vi "Init.vi"(8 "error in (no error)":errorcluster, 11 "Process In":refnum<class "Process.lvclass">) -> (0 "error out":errorcluster, 3 "Process Out":refnum<class "Process.lvclass">)   [LabVIEW 2020, in "Process.lvclass"]
doc: "Initializes the process and creates necessary references. Anything initialized here is released in the Clear.vi method."
uses:
  Process.lvclass
  Protected/Message Cluster.ctl
  Process.lvclass/Process.ctl
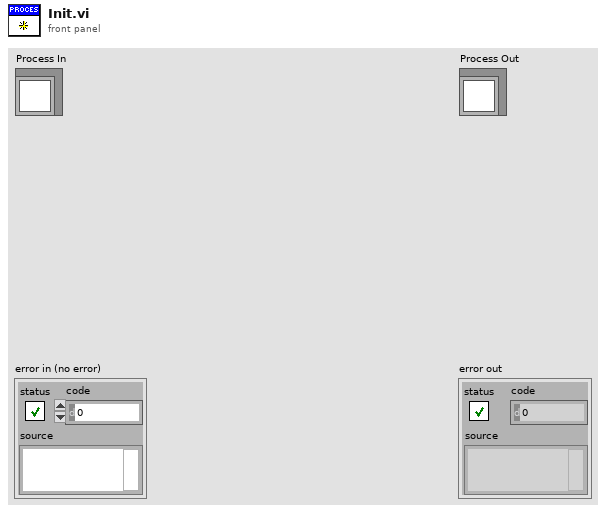
[diagram p1: front panel]
types:
  T1 = typedef "Process.lvclass/Message Cluster.ctl" = cluster{"Message":string, "Message Data":variant}
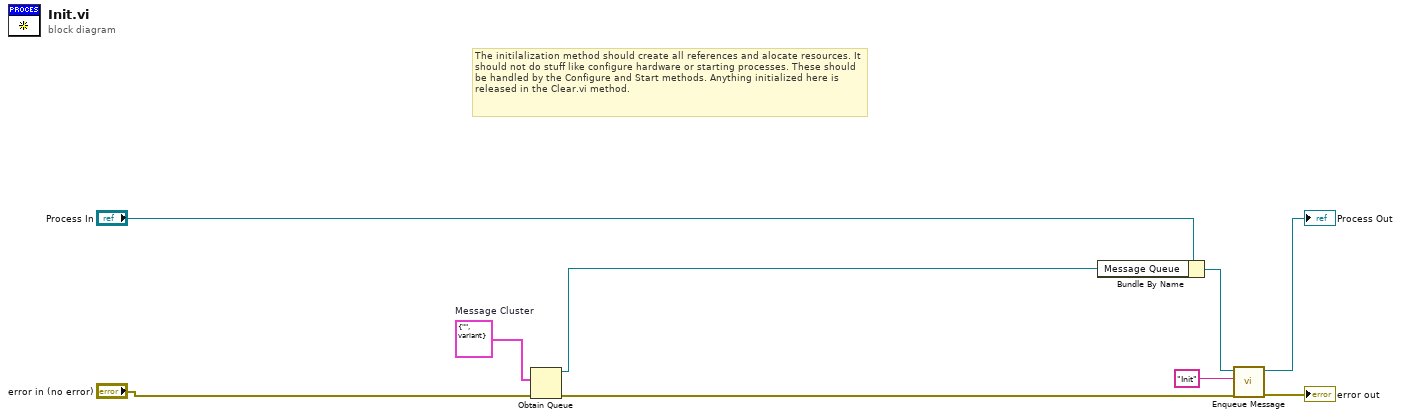
[diagram p0: block diagram]
diagram:
  w1 = T1 {"Message"="", "Message Data"=variant}  # Message Cluster
  # "The initilalization method should create all references and alocate resources. It should not do stuff like configure hardware or starting processes. These should be handled by the Configure and Start methods. Anything initialized here is released in the Clear.vi method."
  n1 = Obtain Queue(element data type=w1, error in (no error)="error in (no error)") -> (queue out=w8:refnum<queue>, error out=w7:errorcluster)  [unwired: 3 in, 1 out]
  n2 = Bundle By Name(cluster="Process In", "Message Queue"=w8) -> (w9:refnum<class "Process.lvclass">)
  n3 = call "Enqueue Message.vi"("error in (no error)"=w7, "Message"="Init", "Process In"=w9) -> ("error out"=→"error out":errorcluster, "Process Out"=→"Process Out":refnum<class "Process.lvclass">)  [unwired: 7 in]
